vi "Grid_Read Status-deleteme.vi"(11 "Grid in":refnum<class "Grid.lvclass">) -> (2 "Grid_Status":cluster{"kW":dbl}, 3 "Grid out":refnum<class "Grid.lvclass">)   [LabVIEW 2015]
uses:
  Grid.lvclass
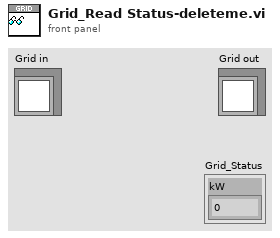
[diagram p1: front panel]
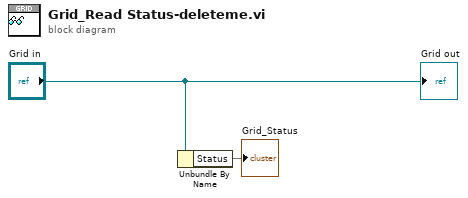
[diagram p0: block diagram]
diagram:
  n1 = Unbundle By Name("Grid in") -> ("Status"=→"Grid_Status")
  "Grid out" <- "Grid in"
